vi "Write Configuration.vi"(8 "error in (no error)":errorcluster, 10 "Configuration":refnum<class "Configuration.lvclass">, 11 "Configuration Interface Test In":refnum<class "Configuration Interface Test.lvclass">) -> (0 "error out":errorcluster, 3 "Configuration Interface Test Out":refnum<class "Configuration Interface Test.lvclass">)   [LabVIEW 2020, in "Configuration Interface Test.lvclass"]
uses:
  Configuration Interface Test.lvclass
  source/Framework/Configuration/Configuration.lvclass
  Configuration Interface Test.lvclass/Configuration Interface Test.ctl
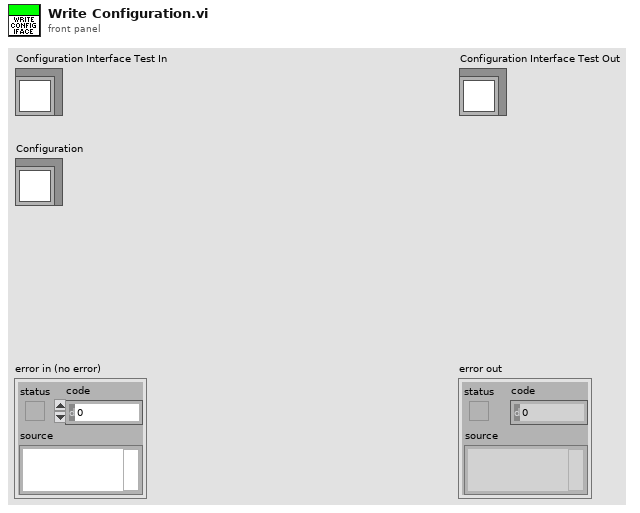
[diagram p1: front panel]
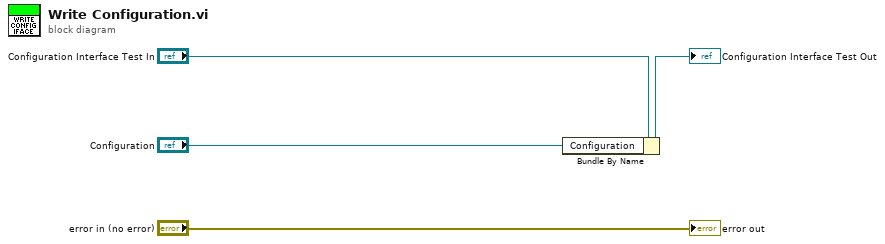
[diagram p0: block diagram]
diagram:
  n1 = Bundle By Name(cluster="Configuration Interface Test In", "Configuration"="Configuration") -> (→"Configuration Interface Test Out":refnum<class "Configuration Interface Test.lvclass">)
  "error out" <- "error in (no error)"
